vi "测试数组截取.vi"() -> ()   [LabVIEW 2019]
panel:
  in  "测试":dbl[](array[numeric])=[5.0, 8.0, 10.0, 15.0]
  in  "字符串":string
  in  "数组 2":dbl[](array[numeric])
  in  "数组":dbl[](array[numeric])
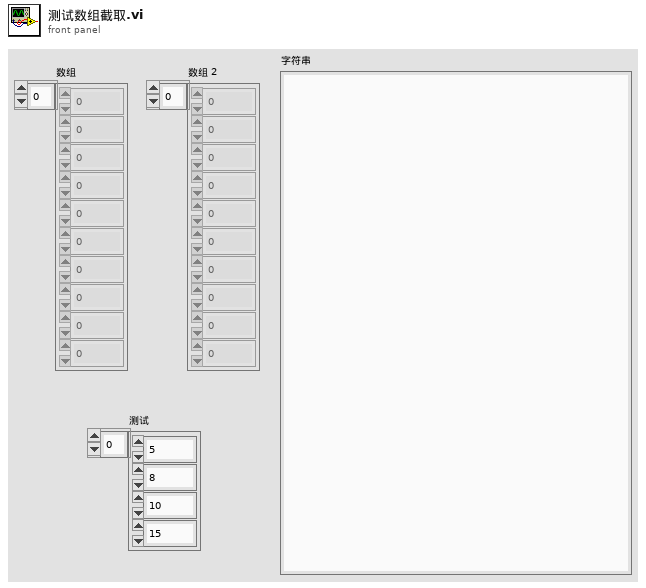
[diagram p1: front panel]
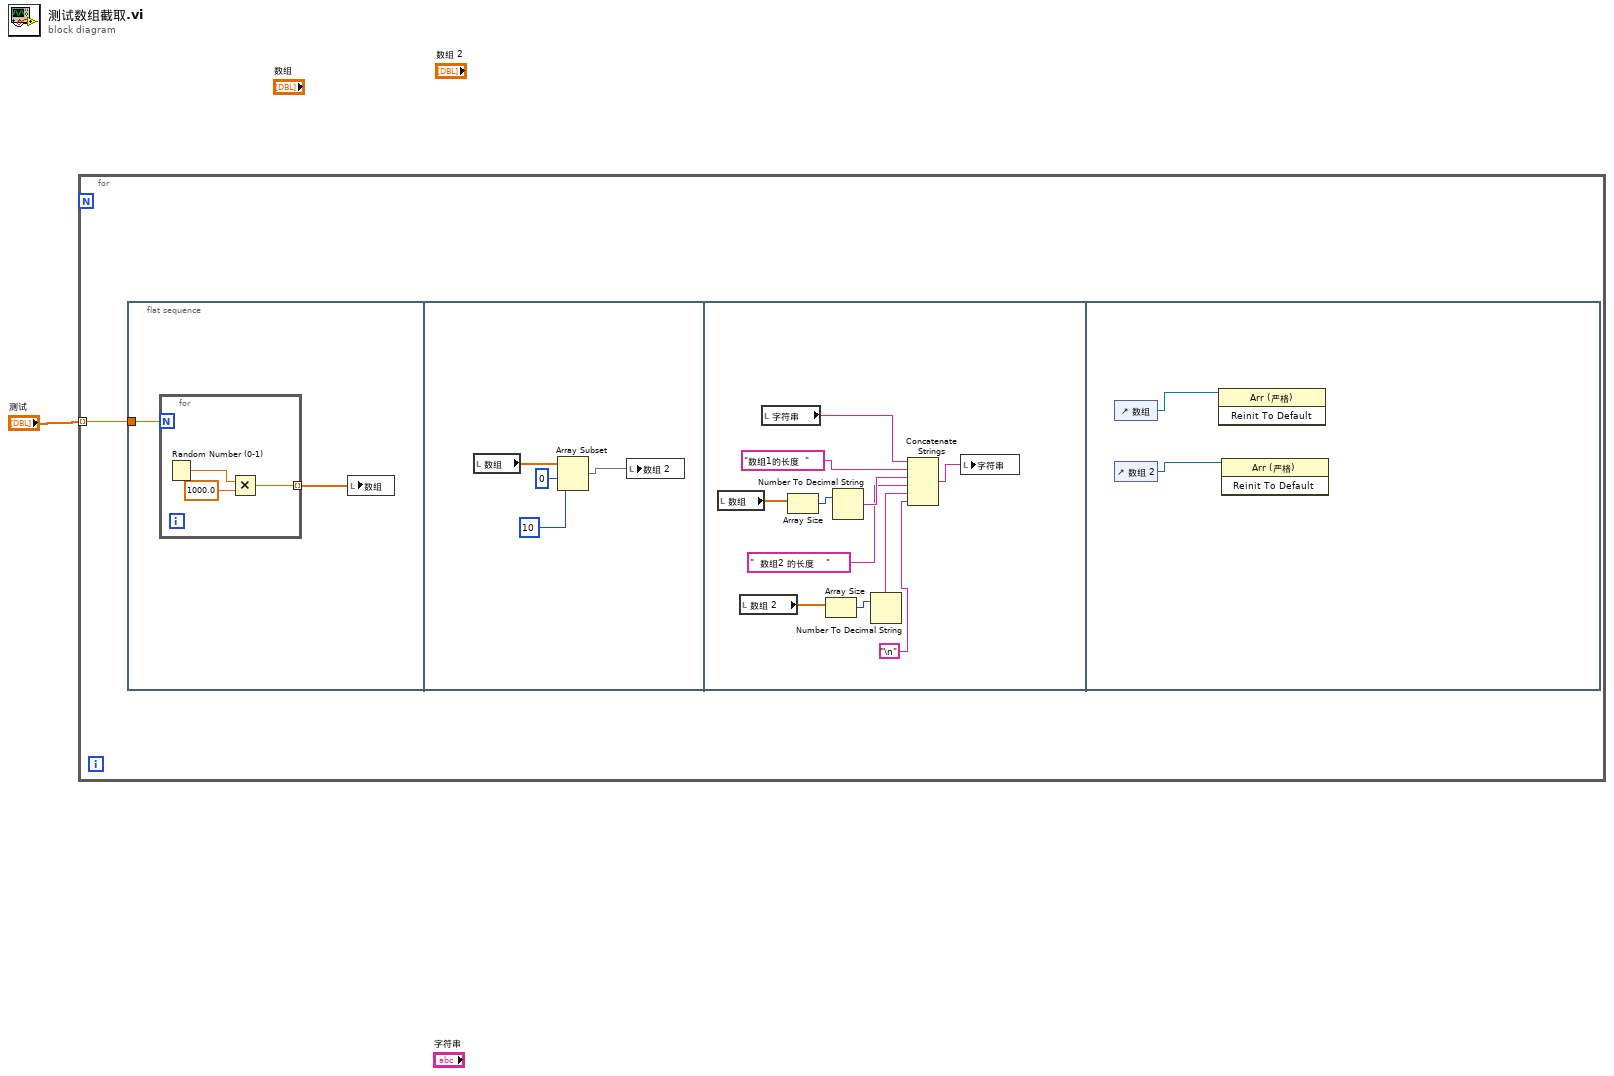
[diagram p0: block diagram]
diagram:
  n1 = for {
    tunnel: "测试" -> [w2] mode=indexing
    n2 = flat-sequence {
      tunnel: w2 -> [w4]
      frame #0 {
        n3 = for {
          N: w4 -> [_]
          tunnel: [w5] -> w3 mode=indexing
          n4 = Random Number (0-1)() -> (number: 0 to 1=w7:dbl)
          n5 = Multiply(x=w7, y=1000.0) -> (x*y=w5:dbl)
        }
        n6 = local write "数组"(w3) -> ()
      }
      frame #1 {
        n7 = local read "数组"() -> (w11:dbl[])
        n8 = Array Subset(array=w11, index=0 ("索引"), length=10 ("长度")) -> (w8:dbl[])
        n9 = local write "数组 2"(w8) -> ()
      }
      frame #2 {
        n10 = local read "数组"() -> (w19:dbl[])
        n11 = local read "数组 2"() -> (w15:dbl[])
        n12 = local read "字符串"() -> (w22:string)
        n13 = Array Size(array=w19) -> (size(s)=w18:i32)
        n14 = Array Size(array=w15) -> (size(s)=w14:i32)
        n15 = Number To Decimal String(number=w18) -> (decimal integer string=w17:string)  [unwired: 1 in]
        n16 = Number To Decimal String(number=w14) -> (decimal integer string=w13:string)  [unwired: 1 in]
        n17 = Concatenate Strings(w22, "数组1的长度  ", w17, "  数组2 的长度    ", w13, "\n") -> (w21:string)
        n18 = local write "字符串"(w21) -> ()
      }
      frame #3 {
        n19 = control-ref of="数组"() -> (w24:refnum<vi>)
        n20 = control-ref of="数组 2"() -> (w23:refnum<vi>)
        n21 = invoke class="Arr (严格)" method="Reinit To Default"(reference=w24) -> ()  [unwired: 2 in, 3 out]
        n22 = invoke class="Arr (严格)" method="Reinit To Default"(reference=w23) -> ()  [unwired: 2 in, 3 out]
      }
    }
  }
